vi "MVP Valve Setup.vi"(8 "error in (no error)":errorcluster, 9 "Baud Rate (9600)":u32(ring)=9600 items=["300"=300, "1200"=1200, "2400"=2400, "9600"=9600], 10 "Number of valves":i32=1, 11 "VISA resource name":refnum<visa-resource-name>="VALVE") -> (0 "error out":errorcluster, 1 "Autoaddressing Output String":string, 2 "Firmware versions":string[](array[string]), 3 "VISA resource name out":refnum<visa-resource-name>)   [LabVIEW 2015]
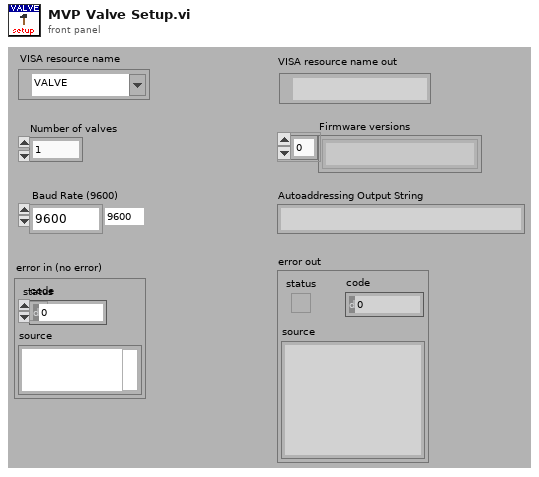
[diagram p1: front panel]
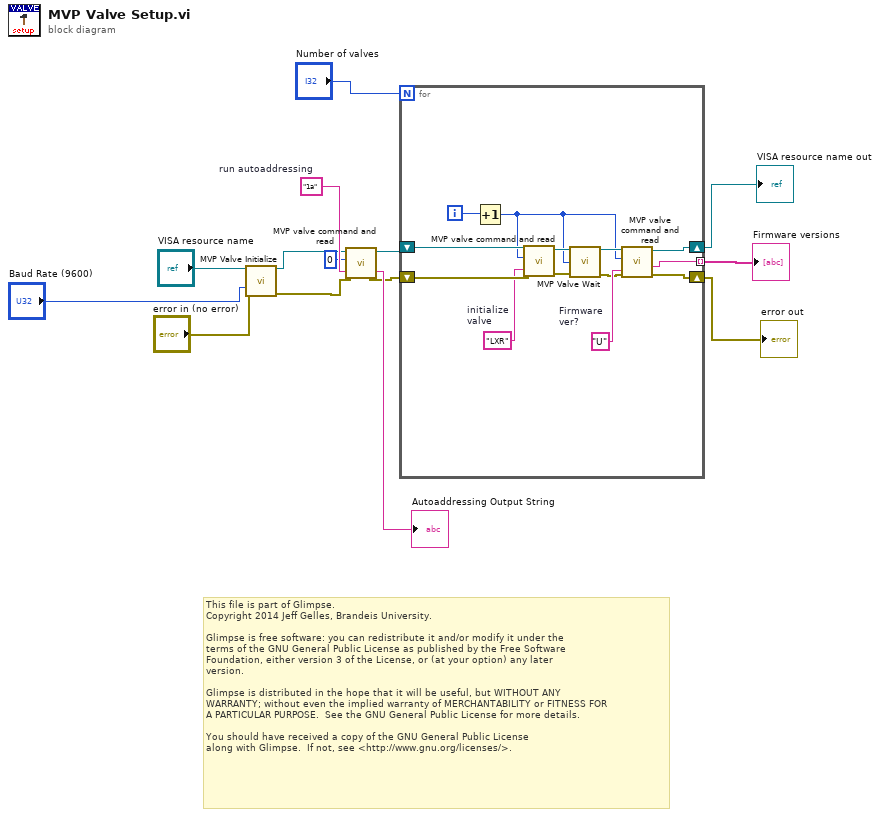
[diagram p0: block diagram]
diagram:
  w12 = "1a"  # run autoaddressing
  # "This file is part of Glimpse. \nCopyright 2014 Jeff Gelles, Brandeis University.    \n\nGlimpse is free software: you can redistribute it and/or modify it under the \nterms of the GNU General Public License as published by the Free Software \nFoundation, either version 3 of the License, or (at your option) any later \nversion.\n\nGlimpse is distributed in the hope that it will be useful, but WITHOUT ANY \nWARRANTY; without even the implied warranty of MERCHANTABILITY or FITNESS FOR \nA PARTICULAR PURPOSE.  See the GNU General Public License for more details.\n\nYou should have received a copy of the GNU General Public License\nalong with Glimpse.  If not, see <http://www.gnu.org/licenses/>."
  n1 = call "MVP Valve Initialize.vi"("VISA resource name"="VISA resource name", "Baud Rate (9600)"="Baud Rate (9600)", "error in (no error)"="error in (no error)") -> ("VISA resource name out"=w11:refnum<visa-resource-name>, "error out"=w10:errorcluster)  [unwired: 11 out]
  n2 = call "MVP valve command and read.vi"("error in"=w10, "command\n(w/o pump # prefix)"=w12, "Valve # (1=a, 2=b, ....  0 = no prefix)"=u8 0, "VISA resource name"=w11) -> ("error out"=w6:errorcluster, "Output String"=→"Autoaddressing Output String":string, "VISA resource name out"=w7:refnum<visa-resource-name>)  [unwired: 2 out]
  n3 = for {
    N: "Number of valves" -> [_]
    shift-right: [w16] -> w3
    shift-left: w6 -> [w26]
    shift-right: [w17] -> w2
    shift-left: w7 -> [w27]
    tunnel: [w15] -> w4 mode=indexing
    i -> [w25]
    w21 = "U"  # Firmware ver?
    w24 = "LXR"  # initialize valve
    n4 = Increment(x=w25) -> (x+1=w18:i32)
    n5 = call "MVP valve command and read.vi"("error in"=w26, "command\n(w/o pump # prefix)"=w24, "Valve # (1=a, 2=b, ....  0 = no prefix)"=w18, "VISA resource name"=w27) -> ("error out"=w23:errorcluster, "VISA resource name out"=w22:refnum<visa-resource-name>)  [unwired: 3 out]
    n6 = call "MVP Valve Wait.vi"("VISA resource name"=w22, "Valve # (1=a, 2=b, ....  0 = no prefix)"=w18, "error in (no error)"=w23) -> ("VISA resource name out"=w19:refnum<visa-resource-name>, "error out"=w20:errorcluster)  [unwired: 11 out]
    n7 = call "MVP valve command and read.vi"("error in"=w20, "command\n(w/o pump # prefix)"=w21, "Valve # (1=a, 2=b, ....  0 = no prefix)"=w18, "VISA resource name"=w19) -> ("error out"=w16:errorcluster, "Output String"=w15:string, "VISA resource name out"=w17:refnum<visa-resource-name>)  [unwired: 2 out]
  }
  "VISA resource name out" <- w2
  "error out" <- w3
  "Firmware versions" <- w4
